vi "pb-stop.vi"(8 "error in (no error)":errorcluster, 11 "path in":path=path "C:/SpinCore/SpinAPI/dll/spinapi64.dll") -> (0 "error out":errorcluster, 3 "path out":path)   [LabVIEW 2018]
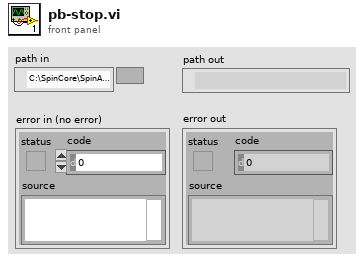
[diagram p1: front panel]
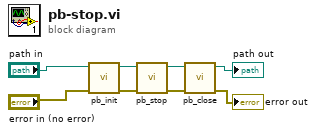
[diagram p0: block diagram]
diagram:
  n1 = call "pb_init.vi"("error in (no error)"="error in (no error)", "path in"="path in") -> ("error out"=w7:errorcluster, "path out"=w8:path)  [unwired: 8 in]
  n2 = call "pb_stop.vi"("error in (no error)"=w7, "path in"=w8) -> ("error out"=w5:errorcluster, "path out"=w6:path)  [unwired: 8 in]
  n3 = call "pb_close.vi"("error in (no error)"=w5, "path in"=w6) -> ("error out"=→"error out":errorcluster, "path out"=→"path out":path)  [unwired: 8 in]
